vi "_RT_CtrlLoop_Pub_Allocator_RS485.vi"() -> ()   [LabVIEW 2018]
uses:
  <vilib>/FPGAPlugInAG/sbRIO-9627/niLvFpga_Close_sbRIO-9627.vi
  <vilib>/FPGAPlugInAG/sbRIO-9627/niLvFpga_Open_sbRIO-9627.vi
  <vilib>/FPGAPlugInAG/sbRIO-9627/niLvFpga_Reset_sbRIO-9627.vi
  <vilib>/FPGAPlugInAG/sbRIO-9627/niLvFpga_Run_sbRIO-9627.vi
  <vilib>/Utility/error.llb/Error Cluster From Error Code.vi
  <vilib>/rvi/errors/niLvFpgaAdjustHostInterfaceError.vi
  <vilib>/rvi/interface/nirviCloseFPGA/nirviCloseFPGA.xnode
  FPGA Bitfiles/ATIQITAnalyser_FPGAZynq7020_FPGAnone.lvbitx
  <vilib>/rvi/interface/nirviOpenFPGA/nirviOpenFPGA.xnode
  <vilib>/rvi/interface/nirviMethod/nirviMethod.xnode
  <vilib>/rvi/interface/nirviReadWriteControl/nirviReadWriteControl.xnode
  NiFpgaLv.dll
panel:
  out "count out":u16
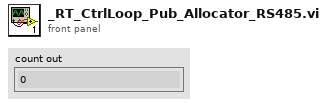
[diagram p1: front panel]
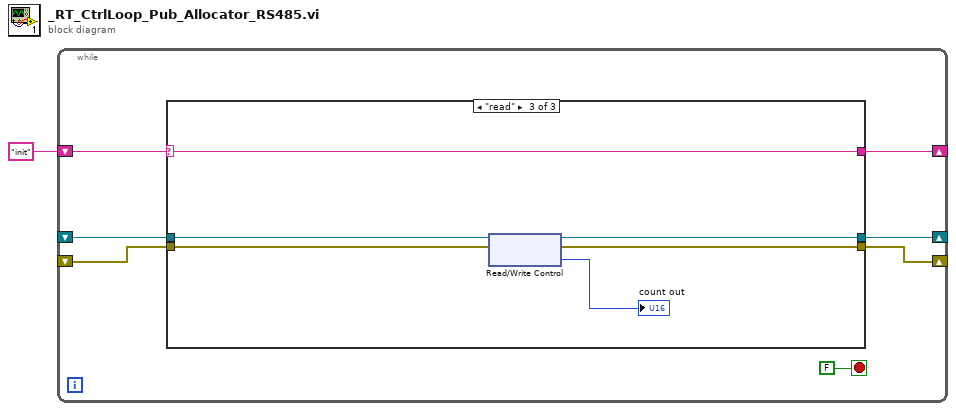
[diagram p0: block diagram]
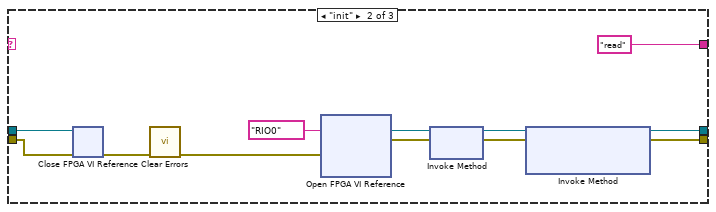
[diagram p3: hidden frame]
diagram:
  n1 = while {
    shift-right: [w7] -> _
    shift-left: _ -> [w8]
    shift-right: [w6] -> _
    shift-left: _ -> [w2]
    shift-right: [w3] -> _
    shift-left: "init" -> [w5]
    stop <- FALSE stop-if-true
    n2 = case shown="\"read\"" w5 {
      selector: w5 -> [w11 _ w29]
      tunnel: w8 -> [w10 w17 w28]
      tunnel: [w10 w16 w26] -> w7
      tunnel: [w9 w15 w27] -> w6
      tunnel: [w11 "read" w29] -> w3
      tunnel: w2 -> [w9 w13 w24]
      frame Default {
      }
      frame "init" {
        n3 = xnode "Close FPGA VI Reference"("FPGA VI Reference In"=w17, "error in"=w13) -> ("error out"=w23:errorcluster)
        n4 = call <vilib>:"Clear Errors.vi"("error in (no error)"=w23) -> ("error out"=w22:errorcluster)  [unwired: 5 in, 1 out]
        n5 = xnode "Open FPGA VI Reference"("error in"=w22, "resource name"=tag "RIO0") -> ("FPGA VI Reference Out"=w21:refnum<k20>, "error out"=w20:errorcluster)
        n6 = xnode "Invoke Method"("FPGA VI Reference In"=w21, "error in"=w20) -> ("FPGA VI Reference Out"=w19:refnum<k20>, "error out"=w18:errorcluster)
        n7 = xnode "Invoke Method"("FPGA VI Reference In"=w19, "error in"=w18) -> ("FPGA VI Reference Out"=w16:refnum<k20>, "error out"=w15:errorcluster)  [unwired: 1 in]
      }
      frame "read" {
        n8 = xnode "Read/Write Control"("FPGA VI Reference In"=w28, "error in"=w24) -> ("FPGA VI Reference Out"=w26:refnum<k20>, "error out"=w27:errorcluster, "count out"=→"count out":u16)
      }
    }
  }
